vi "Reset Buckets.vi"   [LabVIEW 2013]
doc: "Sums up the intensity for pixels within each sector."
uses:
  <vilib>/rvi/Memory/Memory_Emulation/nirvimemoryFastEmulationFpgaImpl.vi
  <instcachedir>/0/nirvimemoryFastEmulationFpgaImpl_5FBAB50466BC4C939F684F8805638BFC.lvgen/nirvimemoryFastEmulationFpgaImpl_5FBAB50466BC4C939F684F8805638BFC_006.vi
  <vilib>/rvi/DataTransferAndStorage/Container/Common/niFpgaContainerGetUniqueNameForEmu.vi
  <vilib>/rvi/Memory/Memory_Emulation/nirvimemoryFastEmulation.vi
  <vilib>/rvi/Memory/Memory_Emulation/nirvimemoryEmulation.vi
  <vilib>/rvi/DataTransferAndStorage/Container/Common/niFpgaContainerExecOnDevCompGetState.vi
  <instcachedir>/0/nirvimemoryFastEmulationFpgaImpl_5FBAB50466BC4C939F684F8805638BFC.lvgen/nirvimemoryFastEmulationFpgaImpl_5FBAB50466BC4C939F684F8805638BFC_007.vi
  <vilib>/rvi/Memory/Memory_Emulation/niFpgaMemoryEmulationCacheClearOnFirstRun.vi
  <vilib>/rvi/Memory/Memory_Emulation/nirvimemoryEmulationManagerCache_MakeExclusive.vi
  <vilib>/rvi/Memory/Memory_Emulation/niFpgaMemoryEmulationValidateCache.vi
  <vilib>/rvi/Memory/Memory_Emulation/nirvimemoryEmulationManagerCache_ReleaseExclusive.vi
  <vilib>/rvi/Memory/Memory_Emulation/nirvimemoryEmulationManagerCache_InsertValue.vi
  <vilib>/Utility/error.llb/Clear Errors.vi
  <vilib>/rvi/Emulation/niFpgaSctlEmulationGetInTimedLoop.vi
  <vilib>/rvi/Memory/Memory_Emulation/nirvimemoryEmulationManagerCache_SetValue.vi
  <vilib>/rvi/Emulation/niFpgaSctlEmulationResourceMgr.vi
  <vilib>/rvi/DataTransferAndStorage/Container/XNode/niFpgaContainer.xnode
  <vilib>/rvi/Memory/Memory_Emulation/niFpgaMemoryEmulationRefIn.vi
types:
  T1 = cluster{"Accumulated Intensity":u32, "Count":u16}
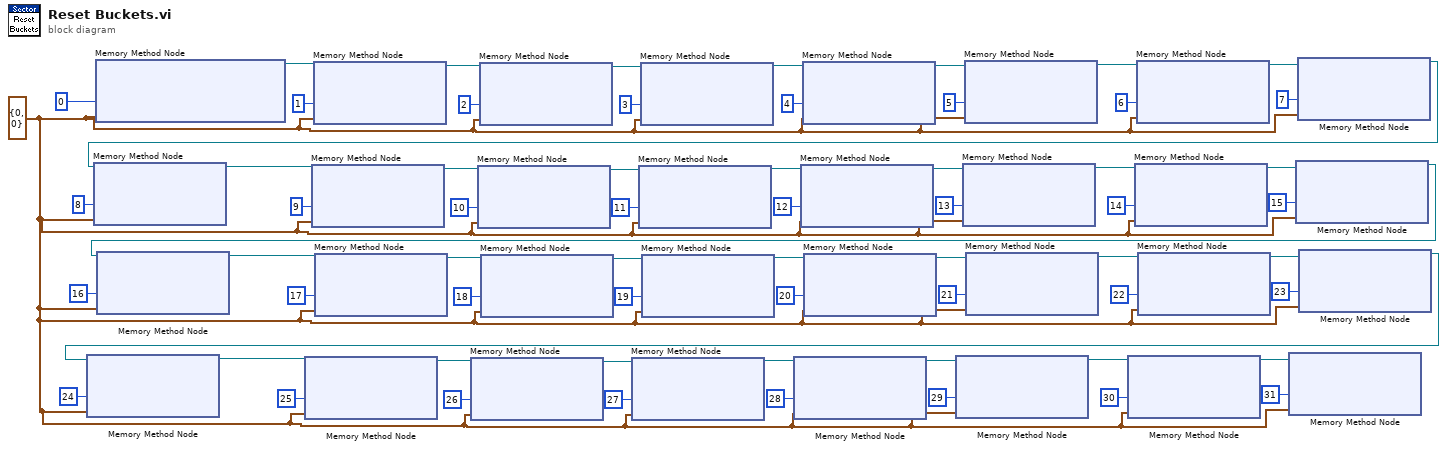
[diagram p0: block diagram]
diagram:
  w1 = T1 {"Accumulated Intensity"=0, "Count"=0} ("Data")
  n1 = xnode ("Memory Method Node")("Address"=u32 0, "Data"=w1) -> ("Memory Out"=w63:refnum<k21>)  [unwired: 1 in]
  n2 = xnode ("Memory Method Node")("Address"=u32 1, "Data"=w1, "Memory In"=w63) -> ("Memory Out"=w60:refnum<k21>)
  n3 = xnode ("Memory Method Node")("Address"=u32 2, "Data"=w1, "Memory In"=w60) -> ("Memory Out"=w58:refnum<k21>)
  n4 = xnode ("Memory Method Node")("Address"=u32 3, "Data"=w1, "Memory In"=w58) -> ("Memory Out"=w56:refnum<k21>)
  n5 = xnode ("Memory Method Node")("Address"=u32 4, "Data"=w1, "Memory In"=w56) -> ("Memory Out"=w54:refnum<k21>)
  n6 = xnode ("Memory Method Node")("Address"=u32 5, "Data"=w1, "Memory In"=w54) -> ("Memory Out"=w52:refnum<k21>)
  n7 = xnode ("Memory Method Node")("Address"=u32 6, "Data"=w1, "Memory In"=w52) -> ("Memory Out"=w50:refnum<k21>)
  n8 = xnode ("Memory Method Node")("Address"=u32 7, "Data"=w1, "Memory In"=w50) -> ("Memory Out"=w34:refnum<k21>)
  n9 = xnode ("Memory Method Node")("Address"=u32 8, "Data"=w1, "Memory In"=w34) -> ("Memory Out"=w36:refnum<k21>)
  n10 = xnode ("Memory Method Node")("Address"=u32 9, "Data"=w1, "Memory In"=w36) -> ("Memory Out"=w39:refnum<k21>)
  n11 = xnode ("Memory Method Node")("Address"=u32 10, "Data"=w1, "Memory In"=w39) -> ("Memory Out"=w41:refnum<k21>)
  n12 = xnode ("Memory Method Node")("Address"=u32 11, "Data"=w1, "Memory In"=w41) -> ("Memory Out"=w43:refnum<k21>)
  n13 = xnode ("Memory Method Node")("Address"=u32 12, "Data"=w1, "Memory In"=w43) -> ("Memory Out"=w45:refnum<k21>)
  n14 = xnode ("Memory Method Node")("Address"=u32 13, "Data"=w1, "Memory In"=w45) -> ("Memory Out"=w47:refnum<k21>)
  n15 = xnode ("Memory Method Node")("Address"=u32 14, "Data"=w1, "Memory In"=w47) -> ("Memory Out"=w49:refnum<k21>)
  n16 = xnode ("Memory Method Node")("Address"=u32 15, "Data"=w1, "Memory In"=w49) -> ("Memory Out"=w18:refnum<k21>)
  n17 = xnode ("Memory Method Node")("Address"=u32 16, "Data"=w1, "Memory In"=w18) -> ("Memory Out"=w32:refnum<k21>)
  n18 = xnode ("Memory Method Node")("Address"=u32 17, "Data"=w1, "Memory In"=w32) -> ("Memory Out"=w29:refnum<k21>)
  n19 = xnode ("Memory Method Node")("Address"=u32 18, "Data"=w1, "Memory In"=w29) -> ("Memory Out"=w27:refnum<k21>)
  n20 = xnode ("Memory Method Node")("Address"=u32 19, "Data"=w1, "Memory In"=w27) -> ("Memory Out"=w25:refnum<k21>)
  n21 = xnode ("Memory Method Node")("Address"=u32 20, "Data"=w1, "Memory In"=w25) -> ("Memory Out"=w23:refnum<k21>)
  n22 = xnode ("Memory Method Node")("Address"=u32 21, "Data"=w1, "Memory In"=w23) -> ("Memory Out"=w21:refnum<k21>)
  n23 = xnode ("Memory Method Node")("Address"=u32 22, "Data"=w1, "Memory In"=w21) -> ("Memory Out"=w19:refnum<k21>)
  n24 = xnode ("Memory Method Node")("Address"=u32 23, "Data"=w1, "Memory In"=w19) -> ("Memory Out"=w2:refnum<k21>)
  n25 = xnode ("Memory Method Node")("Address"=u32 24, "Data"=w1, "Memory In"=w2) -> ("Memory Out"=w4:refnum<k21>)
  n26 = xnode ("Memory Method Node")("Address"=u32 25, "Data"=w1, "Memory In"=w4) -> ("Memory Out"=w7:refnum<k21>)
  n27 = xnode ("Memory Method Node")("Address"=u32 26, "Data"=w1, "Memory In"=w7) -> ("Memory Out"=w9:refnum<k21>)
  n28 = xnode ("Memory Method Node")("Address"=u32 27, "Data"=w1, "Memory In"=w9) -> ("Memory Out"=w11:refnum<k21>)
  n29 = xnode ("Memory Method Node")("Address"=u32 28, "Data"=w1, "Memory In"=w11) -> ("Memory Out"=w13:refnum<k21>)
  n30 = xnode ("Memory Method Node")("Address"=u32 29, "Data"=w1, "Memory In"=w13) -> ("Memory Out"=w15:refnum<k21>)
  n31 = xnode ("Memory Method Node")("Address"=u32 30, "Data"=w1, "Memory In"=w15) -> ("Memory Out"=w17:refnum<k21>)
  n32 = xnode ("Memory Method Node")("Address"=u32 31, "Data"=w1, "Memory In"=w17) -> ()  [unwired: 1 out]
